vi "parseSensorUpdate.vi"(11 "read buffer":string) -> (0 "panic button":bool, 1 "temperature (farenheit)":dbl, 2 "node ID":u8, 3 "parse successful?":bool, 4 "motion sensor":bool, 5 "back door":bool, 6 "front door":bool, 7 "garage door":bool)   [LabVIEW 2011]
panel:
  out "siren":bool
  out "motion sensor power":bool
  out "temperature (celsius)":dbl
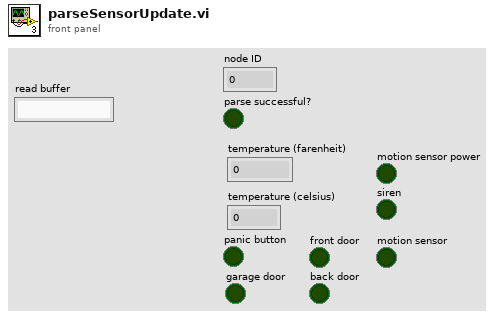
[diagram p1: front panel]
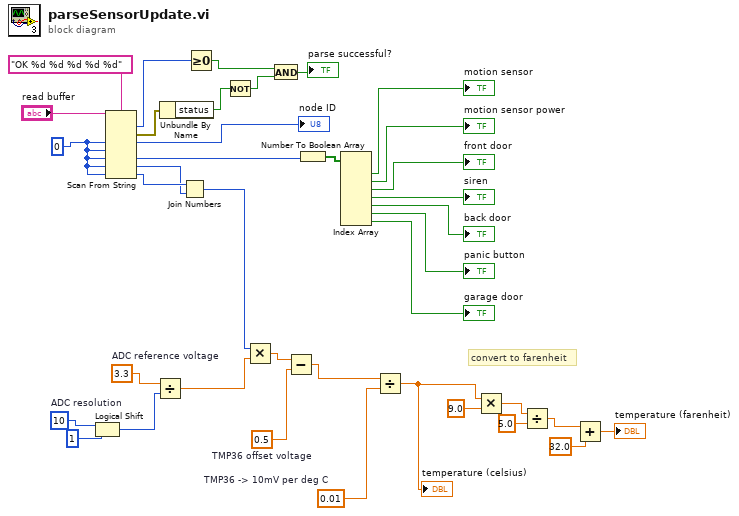
[diagram p0: block diagram]
diagram:
  w24 = 0.01  # TMP36 -> 10mV per deg C
  w26 = 0.5  # TMP36 offset voltage
  w33 = 10  # ADC resolution
  w31 = 3.3  # ADC reference voltage
  w35 = u8 0
  # "convert to farenheit"
  n1 = Logical Shift(y=w33, x=1) -> (x << y=w30:i32)
  n2 = Scan From String(format string="OK %d %d %d %d %d", input string="read buffer", default 1=w35, default 2=w35, default 3=w35, default 4=w35, default 5=w35) -> (offset past scan=w36:u32, error out=w16:errorcluster, output 1=→"node ID":u8, output 3=w3:u8, output 4=w1:u8, output 5=w2:u8)  [unwired: 3 in, 1 out]
  n3 = Divide(x=w31, y=w30) -> (x/y=w28:dbl)
  n4 = Unbundle By Name(w16) -> ("status"=w15:bool)
  n5 = Join Numbers(hi=w2, lo=w1) -> ((hi.lo)=w29:u16)
  n6 = Greater Or Equal To 0?(x=w36) -> (x >= 0?=w14:bool)
  n7 = Not(x=w15) -> (.not. x?=w13:bool)
  n8 = Multiply(x=w29, y=w28) -> (x*y=w27:dbl)
  n9 = And(x=w14, y=w13) -> (x .and. y?=→"parse successful?":bool)
  n10 = Subtract(x=w27, y=w26) -> (x-y=w25:dbl)
  n11 = Number To Boolean Array(number=w3) -> (Boolean array=w11:bool[])
  n12 = Index Array(array=w11) -> (element #1=→"motion sensor":bool, element #2=→"motion sensor power":bool, element #3=→"front door":bool, element #4=→"siren":bool, element #5=→"back door":bool, element #6=→"panic button":bool, element #7=→"garage door":bool)  [unwired: 7 in]
  n13 = Divide(x=w25, y=w24) -> (x/y=w20:dbl)
  "temperature (celsius)" <- w20
  n14 = Multiply(x=w20, y=9.0) -> (x*y=w22:dbl)
  n15 = Divide(x=w22, y=5.0) -> (x/y=w19:dbl)
  n16 = Add(x=w19, y=32.0) -> (x+y=→"temperature (farenheit)":dbl)
